vi "Memory.Pointer.Get Allocated Size.vi"(8 "error in (no error)":errorcluster, 11 "Pointer in":refnum<class "Memory.Pointer.Void.lvclass">) -> (0 "error out":errorcluster, 2 "allocated size":u64 format="%d bytes", 3 "Pointer out":refnum<class "Memory.Pointer.Void.lvclass">)   [LabVIEW 2016, in "LabVIEW Memory Manager.lvlib" / "Memory.Pointer.Void.lvclass"]
uses:
  Memory.Pointer.Void.lvclass
  Memory.Pointer.Void.lvclass/Memory.Pointer.Void.ctl
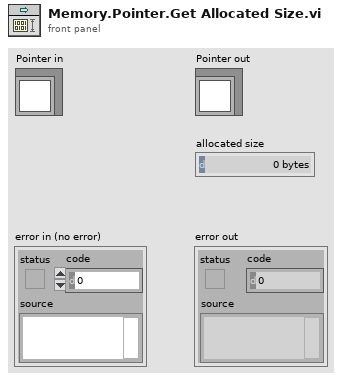
[diagram p1: front panel]
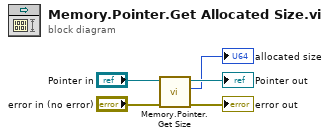
[diagram p0: block diagram]
diagram:
  n1 = call "Memory.Pointer.Get Size.vi"("error in (no error)"="error in (no error)", "Pointer in"="Pointer in") -> ("error out"=→"error out":errorcluster, "size"=→"allocated size":u64, "Pointer out"=→"Pointer out":refnum<class "Memory.Pointer.Void.lvclass">)  [unwired: 7 in]
